vi "Get all Object Items.vi"(8 "error in (no error)":errorcluster, 10 "Offset":i32, 11 "JSON":string) -> (0 "error out":errorcluster, 1 "<JSON>":string[](array[string]) caption="<JSON>Items", 2 "Offset past":i32 caption="Offset past Object", 3 "Item Names":string[](array[string]))   [LabVIEW 2020, in "JSONtext.lvlib"]
doc: "Return all Items in the Object as an array of JSON Values."
uses:
  <vilib>/JDP Science/JSONtext/JSONtext.lvlib
  <vilib>/JDP Science/JSONtext/Parsing/Parsing State.ctl
  <vilib>/JDP Science/JSONtext/Parsing/Advance past Line Ending.vi
  <vilib>/JDP Science/JSONtext/Parsing/Advance past Number.vi
  <vilib>/JDP Science/JSONtext/support/Unescape JSON string.vi
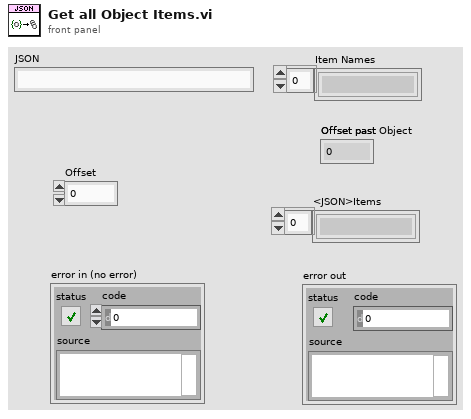
[diagram p1: front panel]
types:
  T1 = typedef "JSONtext.lvlib/Parsing State.ctl" = enum16{"Parser Error", "Object", "Array", "String", "Number/Other", "Leading Whitespace", "Object end", "Array end", "Value end"}
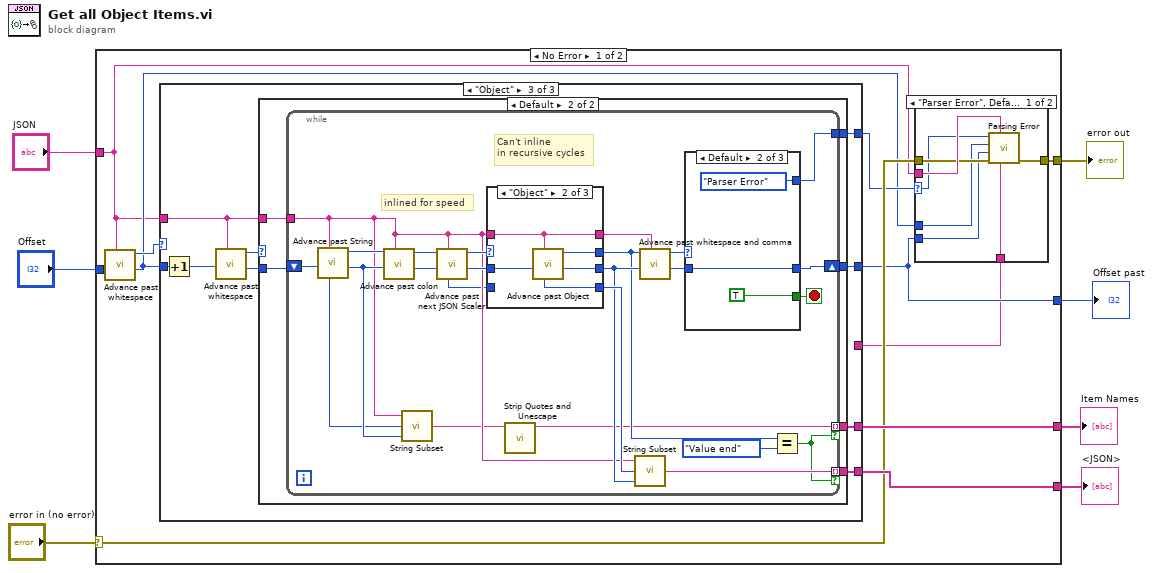
[diagram p0: block diagram]
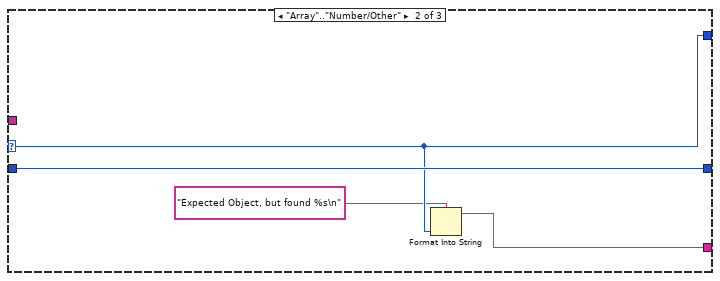
[diagram p3: hidden frame]
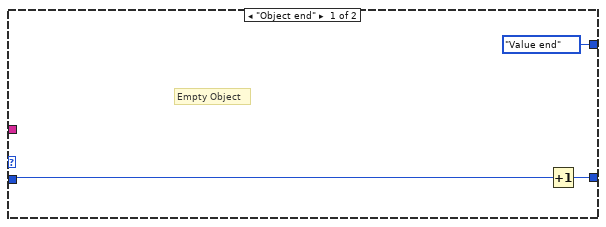
[diagram p4: hidden frame]
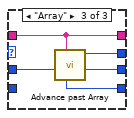
[diagram p6: hidden frame]
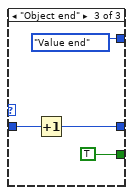
[diagram p8: hidden frame]
diagram:
  n1 = case shown="No Error" "error in (no error)" {
    selector: "error in (no error)" -> [w13 w98]
    tunnel: [w18 _] -> w7
    tunnel: [w17 _] -> w6
    tunnel: "Offset" -> [w16 w97]
    tunnel: [w14 w98] -> w4
    tunnel: [w12 w97] -> w2
    tunnel: "JSON" -> [w9 _]
    frame No Error {
      n2 = call <vilib>:"Advance past whitespace.vi"("JSON"=w9, "Offset"=w16) -> ("Offset of first non-whitespace"=w10:i32, "Parser State"=w15:T1)  [unwired: 7 in, 1 out]
      n3 = case shown="\"Object\"" w15 {
        selector: w15 -> [w20 w22 _]
        tunnel: [w20 w22 w33] -> w11
        tunnel: [_ _ w32] -> w18
        tunnel: [_ _ w31] -> w17
        tunnel: w10 -> [w19 w24 w30]
        tunnel: w9 -> [_ _ w26]
        tunnel: [w19 w24 w29] -> w12
        tunnel: [_ w23 _] -> w8
        frame "Parser Error", Default {
        }
        frame "Array".."Number/Other" {
          n4 = Format Into String(format string="Expected Object, but found %s\n", w22) -> (resulting string=w23:string)  [unwired: 2 in, 1 out]
        }
        frame "Object" {
          n5 = Increment(x=w30) -> (x+1=w28:i32)
          n6 = call <vilib>:"Advance past whitespace.vi"("JSON"=w26, "Offset"=w28) -> ("Offset of first non-whitespace"=w27:i32, "Parser State"=w25:T1)  [unwired: 7 in, 1 out]
          n7 = case shown="Default" w25 {
            tunnel: [Parsing_State."Value end" w42] -> w33
            tunnel: [_ w41] -> w32
            tunnel: [_ w40] -> w31
            tunnel: [w35 w39] -> w29
            tunnel: w27 -> [w34 w38]
            tunnel: w26 -> [_ w37]
            frame "Object end" {
              # "Empty Object"
              n8 = Increment(x=w34) -> (x+1=w35:i32)
            }
            frame Default {
              n9 = while {
                shift-right: [w63] -> w39
                shift-left: w38 -> [w43]
                tunnel: w37 -> [w52]
                tunnel: [w61] -> w42
                tunnel: [w46] -> w41 mode=indexing if=w48
                tunnel: [w51] -> w40 mode=indexing if=w48
                stop <- w62 stop-if-true
                # "Can't inline\nin recursive cycles"
                # "inlined for speed"
                n10 = call <vilib>:"Advance past String.vi"("JSON"=w52, "Offset"=w43) -> ("Offset past match"=w55:i32, "State"=w66:T1, "Value start out"=w45:i32)  [unwired: 7 in]
                n11 = call <vilib>:"Advance past colon.vi"("JSON"=w52, "Offset"=w55, "State"=w66) -> ("index"=w57:i32, "State"=w58:T1)  [unwired: 7 in]
                n12 = call <vilib>:"String Subset.vi"("Offset past End"=w55, "Start offset"=w45, "JSON"=w52) -> ("substring"=w47:string)  [unwired: 2 in]
                n13 = call <vilib>:"Advance past next JSON Scaler.vi"("JSON"=w52, "Offset"=w57, "Parser State in"=w58) -> ("Offset Past"=w56:i32, "Parser State"=w59:T1, "Value start"=w44:i32)  [unwired: 6 in]
                n14 = case shown="\"Object\"" w59 {
                  selector: w59 -> [w69 _ _]
                  tunnel: w56 -> [w68 w75 w80]
                  tunnel: [w69 w74 w79] -> w50
                  tunnel: [w68 w73 w78] -> w53
                  tunnel: w52 -> [w70 w72 w77]
                  tunnel: [w70 w72 w77] -> w60
                  tunnel: [w67 w71 w76] -> w54
                  tunnel: w44 -> [w67 _ _]
                  frame Default {
                  }
                  frame "Object" {
                    n15 = call <vilib>:"Advance past Object.vi"("JSON"=w72, "Offset"=w75) -> ("Offset past Object"=w73:i32, "State"=w74:T1, "Object Start"=w71:i32)  [unwired: 7 in]
                  }
                  frame "Array" {
                    n16 = call <vilib>:"Advance past Array.vi"("JSON"=w77, "Offset"=w80) -> ("Offset past Array"=w78:i32, "State"=w79:T1, "Array Start"=w76:i32)  [unwired: 6 in, 1 out]
                  }
                }
                n17 = call <vilib>:"Strip Quotes and Unescape.vi"("String"=w47) -> ("result string"=w46:string)  [unwired: 9 in, 1 out]
                n18 = call <vilib>:"String Subset.vi"("Offset past End"=w53, "Start offset"=w54, "JSON"=w52) -> ("substring"=w51:string)  [unwired: 2 in]
                n19 = call <vilib>:"Advance past whitespace and comma.vi"("JSON"=w60, "Offset"=w53, "State in"=w50) -> ("Offset past match"=w65:i32, "State"=w64:T1)  [unwired: 6 in, 1 out]
                n20 = case shown="Default" w64 {
                  tunnel: [_ TRUE TRUE] -> w62
                  tunnel: [_ Parsing_State."Parser Error" Parsing_State."Value end"] -> w61
                  tunnel: w65 -> [w81 w82 w86]
                  tunnel: [w81 w82 w85] -> w63
                  frame "Object".."Number/Other" {
                  }
                  frame Default {
                  }
                  frame "Object end" {
                    n21 = Increment(x=w86) -> (x+1=w85:i32)
                  }
                }
                n22 = Equal?(x=w50, y=Parsing_State."Value end") -> (x = y?=w48:bool)
              }
            }
          }
        }
      }
      n23 = case shown="\"Parser Error\", Default" w11 {
        selector: w11 -> [w90 _]
        tunnel: w9 -> [w95 _]
        tunnel: w13 -> [w94 w96]
        tunnel: [w93 w96] -> w14
        tunnel: w10 -> [w92 _]
        tunnel: w12 -> [w91 _]
        tunnel: w8 -> [w89 _]
        frame "Parser Error", Default {
          n24 = call <vilib>:"Parsing Error.vi"("initial string"=w89, "JSON"=w95, "error in (no error)"=w94, "Offset past match"=w91, "Value start"=w92, "State"=w90) -> ("error out"=w93:errorcluster)  [unwired: 5 in]
        }
        frame "Value end" {
        }
      }
    }
    frame Error {
    }
  }
  "Item Names" <- w7
  "<JSON>" <- w6
  "error out" <- w4
  "Offset past" <- w2
